vi "Show_GUI.vi"(8 "error in (no error)":errorcluster caption="entrée d'erreur (pas d'erreur)", 10 "Show_GUI":bool=TRUE, 11 "Actor_EventStart en entrée":refnum<class "Actor_EventStart.lvclass">) -> (0 "error out":errorcluster caption="sortie d'erreur", 3 "Actor_EventStart en sortie":refnum<class "Actor_EventStart.lvclass">)   [LabVIEW 2020, in "Library Core.lvlib" / "Actor_EventStart.lvlib" / "Actor_EventStart.lvclass"]
uses:
  Actor_EventStart.lvclass
  Commun VI/TypeDef/Variable Printable.ctl
  Actor_EventStart.lvclass/Actor_EventStart.ctl
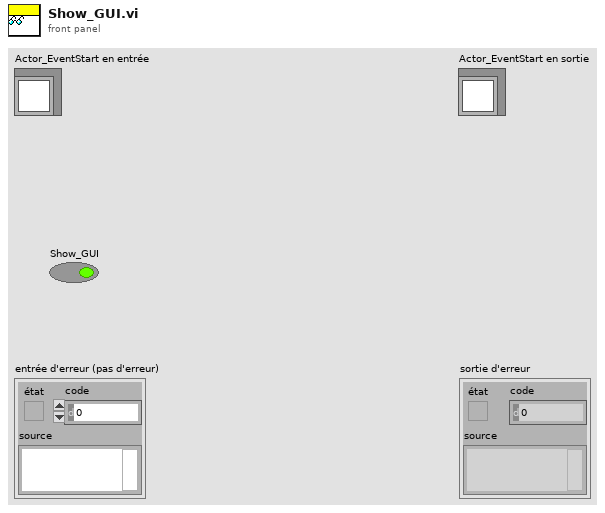
[diagram p1: front panel]
types:
  T1 = enum16{"Get Variable", "Get All Variables", "Set Variable", "Delete Variable", "Delete All Variable"}
  T2 = typedef "Variable Printable.ctl" = string
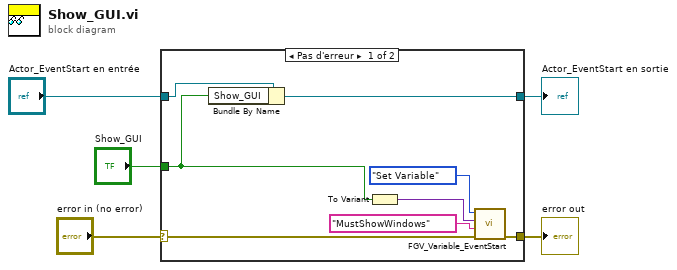
[diagram p0: block diagram]
diagram:
  n1 = case shown="Pas d'erreur" "error in (no error)" {
    selector: "error in (no error)" -> [w7 w14]
    tunnel: [w6 w14] -> w4
    tunnel: [w13 w15] -> w2
    tunnel: "Actor_EventStart en entrée" -> [w12 w15]
    tunnel: "Show_GUI" -> [w10 _]
    frame No Error {
      n2 = Bundle By Name(cluster=w12, "Show_GUI"=w10) -> (w13:refnum<class "Actor_EventStart.lvclass">)
      n3 = To Variant(anything=w10) -> (Variant=w9:variant)
      n4 = call "FGV_Variable_EventStart.vi"("error in (no error)"=w7, "Variable"=T2 "MustShowWindows", "Data In"=w9, "Function"=T1."Set Variable") -> ("error out"=w6:errorcluster)  [unwired: 5 in, 2 out]
    }
    frame Error {
    }
  }
  "error out" <- w4
  "Actor_EventStart en sortie" <- w2
